vi "Pack Connection Handler.vi"(4 "State Change Callback":refnum<class "IConnectionStateChangeCallback.lvclass">, 5 "PersistantConnectionHandler in":refnum<class "PersistantConnectionHandler.lvclass">, 6 "Message Return Policy":refnum<class "IMessageReturnPolicy.lvclass">, 7 "Log Alias":string, 8 "Write Strategy":refnum<class "IWriteStrategy.lvclass">, 9 "Read Strategy":refnum<class "IReadStrategy.lvclass">, 10 "Connection Factory Type":refnum<class "IConnectionFactory.lvclass">, 11 "Log Instance":refnum<class "LoggerReference.lvclass">) -> (3 "PersistantConnectionHandler out":refnum<class "PersistantConnectionHandler.lvclass">)   [LabVIEW 2019, in "PersitantConnectionHandler.lvlib" / "PersistantConnectionHandler.lvclass"]
uses:
  <vilib>/gpm_packages/@cs/Network-interface/Source/PersistantConnectionHandler/PersistantConnectionHandler/PersistantConnectionHandler.lvclass
  C:/Program Files/National Instruments/LabVIEW 2019/vi.lib/gpm_packages/@cs/Network-interface/Source/Logged Actor/LoggedActor.lvclass
  <vilib>/gpm_packages/@cs/event-logger/Source/Composed Log/LoggerReference/LoggerReference.lvclass
  <vilib>/gpm_packages/@cs/Network-interface/Source/MessagingInterfaces/IReadStrategy/IReadStrategy.lvclass
  <vilib>/gpm_packages/@cs/Network-interface/Source/MessagingInterfaces/IWriteStrategy/IWriteStrategy.lvclass
  <vilib>/gpm_packages/@cs/Network-interface/Source/IConnectionFactory/IConnectionFactory.lvclass
  <vilib>/gpm_packages/@cs/Network-interface/Source/MessagingInterfaces/IMessageReturnPolicy/IMessageReturnPolicy.lvclass
  <vilib>/gpm_packages/@cs/Network-interface/Source/MessagingInterfaces/IConnectionStateChangeCallback/IConnectionStateChangeCallback.lvclass
  <vilib>/gpm_packages/@cs/Network-interface/Source/PersistantConnectionHandler/PersistantConnectionHandler/PersistantConnectionHandler.lvclass/PersistantConnectionHandler.ctl
  <vilib>/gpm_packages/@cs/Network-interface/Source/Logged Actor/LoggedActor.lvclass/LoggedActor.ctl
  <vilib>/gpm_packages/@cs/Network-interface/Source/Logged Actor/LoggedActor.lvclass
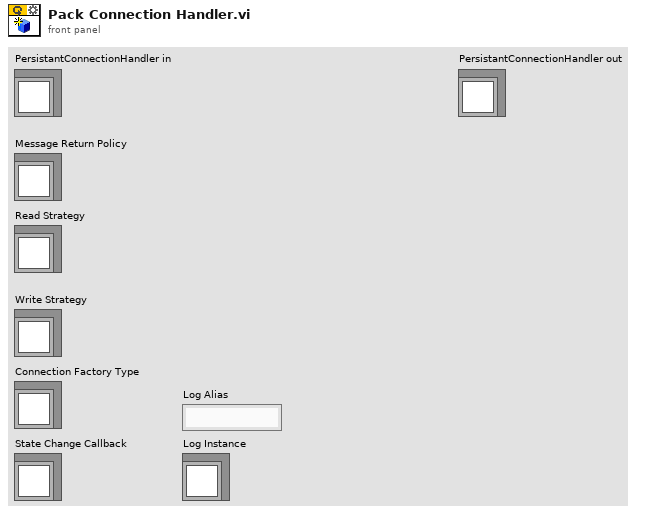
[diagram p1: front panel]
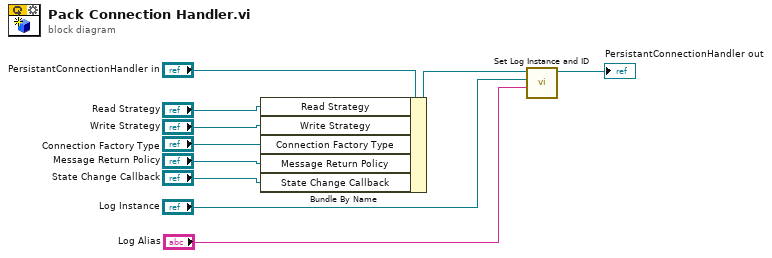
[diagram p0: block diagram]
diagram:
  n1 = Bundle By Name(cluster="PersistantConnectionHandler in", "Read Strategy"="Read Strategy", "Write Strategy"="Write Strategy", "Connection Factory Type"="Connection Factory Type", "Message Return Policy"="Message Return Policy", "State Change Callback"="State Change Callback") -> (w9:refnum<class "PersistantConnectionHandler.lvclass">)
  n2 = call <vilib>:"Set Log Instance and ID.vi"("Log Alias"="Log Alias", "Log Instance"="Log Instance", "LoggedActor in"=w9) -> ("LoggedActor out"=→"PersistantConnectionHandler out":refnum<class "PersistantConnectionHandler.lvclass">)  [unwired: 8 in]
